vi "Configure Measurement (Swept SA).vi"(0 "VISA resource name":refnum<visa-resource-name>, 1 "Enable N dB Points (F: Disable)":bool, 2 "N dB Value (-3.01dB)":dbl=-3.01, 5 "Phase Noise Operation (0: Auto)":i32(ring) items=["Auto", "Offset < 20 kHz", "Offset > 30 kHz", "Fast Tuning"], 7 "ADC Dither (0: Auto)":i32(ring) items=["Auto", "On", "Off"], 9 "Filter Bandwidth (0: -3dB)":i32(ring) items=["-3dB", "-6dB", "Noise", "Impulse"], 11 "error in (no error)":errorcluster, 12 "Bandwidth Filter Type (0: Gaussian)":i32(ring) items=["Gaussian", "Flattop"]) -> (4 "VISA resource name out":refnum<visa-resource-name>, 15 "error out":errorcluster)   [LabVIEW 2018, in "Agilent MXA Series.lvlib"]
doc: "Sets the Swept SA measurement parameters."
uses:
  Agilent MXA Series.lvlib
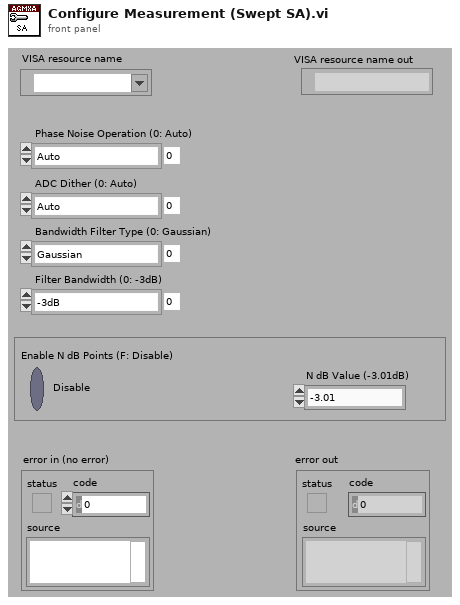
[diagram p1: front panel]
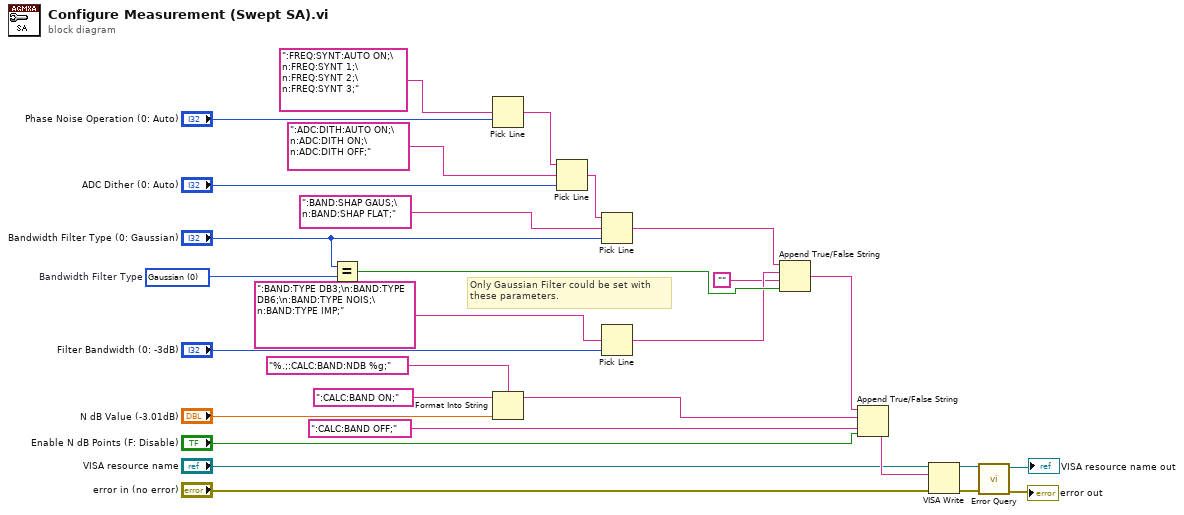
[diagram p0: block diagram]
diagram:
  w1 = 0 items=["Gaussian", "Flattop"]  # Bandwidth Filter Type
  # "Only Gaussian Filter could be set with \nthese parameters."
  n1 = Equal?(x="Bandwidth Filter Type (0: Gaussian)", y=w1) -> (x = y?=w6:bool)
  n2 = Pick Line(multi-line string=":FREQ:SYNT:AUTO ON;\n:FREQ:SYNT 1;\n:FREQ:SYNT 2;\n:FREQ:SYNT 3;" ("Phase Noise Operation"), line index="Phase Noise Operation (0: Auto)") -> (output string=w25:string)  [unwired: 1 in]
  n3 = Format Into String(format string="%.;:CALC:BAND:NDB %g;", initial string=":CALC:BAND ON;", "N dB Value (-3.01dB)") -> (resulting string=w17:string)  [unwired: 1 in, 1 out]
  n4 = Pick Line(string ("")=w25, multi-line string=":ADC:DITH:AUTO ON;\n:ADC:DITH ON;\n:ADC:DITH OFF;", line index="ADC Dither (0: Auto)") -> (output string=w15:string)
  n5 = Pick Line(string ("")=w15, multi-line string=":BAND:SHAP GAUS;\n:BAND:SHAP FLAT;", line index="Bandwidth Filter Type (0: Gaussian)") -> (output string=w7:string)
  n6 = Pick Line(multi-line string=":BAND:TYPE DB3;\n:BAND:TYPE DB6;\n:BAND:TYPE NOIS;\n:BAND:TYPE IMP;", line index="Filter Bandwidth (0: -3dB)") -> (output string=w5:string)  [unwired: 1 in]
  n7 = Append True/False String(1:w6, 2:"", 3:w5, 4:w7) -> (0:w3:string)
  n8 = Append True/False String(1:"Enable N dB Points (F: Disable)", 2:":CALC:BAND OFF;" ("false string"), 3:w17, 4:w3) -> (0:w14:string)
  n9 = VISA Write(VISA resource name="VISA resource name", write buffer=w14, error in (no error)="error in (no error)") -> (VISA resource name out=w11:refnum<visa-resource-name>, error out=w10:errorcluster)  [unwired: 1 out]
  n10 = call "Error Query.vi"("error in (no error)"=w10, "VISA resource name"=w11) -> ("error out"=→"error out":errorcluster, "VISA resource name out"=→"VISA resource name out":refnum<visa-resource-name>)  [unwired: 6 in, 2 out]
